vi "Sine Wave Test UI.vi"() -> ()   [LabVIEW 2015]
uses:
  Sub VIs/Actions.ctl
  Sub VIs/UI Refs.ctl
panel:
  in  "Help":bool
  in  "Settings":bool
  in  "Acquire":bool
  in  "Save":bool
  in  "Print":bool
  in  "Collapse Left":bool
  out "System Waveform Graph":dynamicdata(graph)=[{"t0"=timestamp(0 s since 1904-01-01), "dt"=0.001, "Y"=[-0.05212445512283584, -0.13336150644145808, 0.09686939475676047, 0.04269824059040653, 0.408386715636668, 0.1440963615851781, 0.18338040046154938, 0.5892398993428211, 0.2874755098028772, 0.42360867723351825, 0.39872198705884654, 0.49492986038483694, 0.8476469048510542, 0.5502130098060466, 0.7615388502014413, 0.6858061725246473, 0.765626496308488, 0.759950609248319, 0.913326650050298, 0.9293117069210004, 0.800454971802382, 0.9582885119713533, 1.033746579420675, 1.1831812892834357, 1.131684751301113, 1.1552984321319346, 0.9307610879266989, 1.0357903353668672, 0.7799760446349399, 0.9991309011630207, 0.9067651709329292, 0.9151844666347541, 0.7255708379595651, 0.7577153828467509, 0.76888934319496, 0.8791263479599363, 0.573195316103824, 0.82990628981861, 0.7959395065048407, 0.5455011585933895, 0.4133382261196344, 0.6023069220593702, 0.5471975645283245, 0.5729824629790687, 0.32581411586728487, 0.4323793250489525, 0.13206589194170887, 0.1566622503107214, 0.1943338680098371, -0.04642694048796602, -0.2187165688160441, -0.20901733138094658, 0.007409387766718373, -0.0945831190430492, -0.43328760979874337, -0.25787051409192135, -0.35671739178910694, -0.547611159639428, -0.7119832109077749, -0.6863088159770322, -0.7090502155660231, -0.7901918000137165, -0.6345319422588895, -0.8506202480018857, -0.952891386251698, -0.8864875433466509, -0.8104299150902663, -0.9655915717801792, -0.8044911508280994, -1.0556240415291098, -1.0702070678506619, -1.0265709175924453, -0.9505910211913751, -0.8618792724066139, -0.8436551316564458, -1.1601036667952578, -0.8804024988738188, -0.9488727250175957, -1.0109560414740402, -0.8017015754829107, -0.7668685893134745, -0.893413883311738, -0.7879424291614304, -0.8969827648567197, -0.6349738094147083, -0.592324080467644, -0.5406421151081083, -0.5744385812404026, -0.5106203917953414, -0.5414315844140066, -0.6483405504809772, -0.4993822273028547, -0.6243011215873379, -0.2714483922916202, -0.12038060671565365, -0.19885740767232296, -0.3350758453632484, -0.055660662182264856, -0.1953685024576336, -0.06497850198814607], "attributes"=variant("NI_ChannelName"=variant(string "Sine with Uniform Noise"), "NI_ExpIsRelativeTime"=variant(bool TRUE), "NI_ExpStartTimeStamp"=variant(timestamp timestamp(3347556890.3866034 s since 1904-01-01)), "NI_ExpTimeStamp"=variant(timestamp timestamp(3347556890.3866034 s since 1904-01-01)), "NI_ExpXDimension"=variant(string "t"))}, {"t0"=timestamp(0 s since 1904-01-01), "dt"=0.001, "Y"=[nan, nan, nan, nan, nan, nan, nan, nan, nan, nan, nan, nan, nan, nan, nan, nan, nan, nan, nan, nan, nan, nan, 1.033746579420675, 1.1831812892834357, 1.131684751301113, 1.1552984321319346, nan, 1.0357903353668672, nan, nan, nan, nan, nan, nan, nan, nan, nan, nan, nan, nan, nan, nan, nan, nan, nan, nan, nan, nan, nan, nan, nan, nan, nan, nan, nan, nan, nan, nan, nan, nan, nan, nan, nan, nan, nan, nan, nan, nan, nan, -1.0556240415291098, -1.0702070678506619, -1.0265709175924453, nan, nan, nan, -1.1601036667952578, nan, nan, -1.0109560414740402, nan, nan, nan, nan, nan, nan, nan, nan, nan, nan, nan, nan, nan, nan, nan, nan, nan, nan, nan, nan, nan], "attributes"=variant("NI_ChannelName"=variant(string "Failures"))}, {"t0"=timestamp(0 s since 1904-01-01), "dt"=0.001, "Y"=[1.0, 1.0, 1.0, 1.0, 1.0, 1.0, 1.0, 1.0, 1.0, 1.0, 1.0, 1.0, 1.0, 1.0, 1.0, 1.0, 1.0, 1.0, 1.0, 1.0, 1.0, 1.0, 1.0, 1.0, 1.0, 1.0, 1.0, 1.0, 1.0, 1.0, 1.0, 1.0, 1.0, 1.0, 1.0, 1.0, 1.0, 1.0, 1.0, 1.0, 1.0, 1.0, 1.0, 1.0, 1.0, 1.0, 1.0, 1.0, 1.0, 1.0, 1.0, 1.0, 1.0, 1.0, 1.0, 1.0, 1.0, 1.0, 1.0, 1.0, 1.0, 1.0, 1.0, 1.0, 1.0, 1.0, 1.0, 1.0, 1.0, 1.0, 1.0, 1.0, 1.0, 1.0, 1.0, 1.0, 1.0, 1.0, 1.0, 1.0, 1.0, 1.0, 1.0, 1.0, 1.0, 1.0, 1.0, 1.0, 1.0, 1.0, 1.0, 1.0, 1.0, 1.0, 1.0, 1.0, 1.0, 1.0, 1.0, 1.0], "attributes"=variant("NI_ChannelName"=variant(string "Upper Limit"))}, {"t0"=timestamp(0 s since 1904-01-01), "dt"=0.001, "Y"=[-1.0, -1.0, -1.0, -1.0, -1.0, -1.0, -1.0, -1.0, -1.0, -1.0, -1.0, -1.0, -1.0, -1.0, -1.0, -1.0, -1.0, -1.0, -1.0, -1.0, -1.0, -1.0, -1.0, -1.0, -1.0, -1.0, -1.0, -1.0, -1.0, -1.0, -1.0, -1.0, -1.0, -1.0, -1.0, -1.0, -1.0, -1.0, -1.0, -1.0, -1.0, -1.0, -1.0, -1.0, -1.0, -1.0, -1.0, -1.0, -1.0, -1.0, -1.0, -1.0, -1.0, -1.0, -1.0, -1.0, -1.0, -1.0, -1.0, -1.0, -1.0, -1.0, -1.0, -1.0, -1.0, -1.0, -1.0, -1.0, -1.0, -1.0, -1.0, -1.0, -1.0, -1.0, -1.0, -1.0, -1.0, -1.0, -1.0, -1.0, -1.0, -1.0, -1.0, -1.0, -1.0, -1.0, -1.0, -1.0, -1.0, -1.0, -1.0, -1.0, -1.0, -1.0, -1.0, -1.0, -1.0, -1.0, -1.0, -1.0], "attributes"=variant("NI_ChannelName"=variant(string "Lower Limit"))}]
  in  "Collapse Right":bool
  out "Table Control":string[][](table)=[["12/31/1903 6:00:00 PM", "-0.052"], ["12/31/1903 6:00:00 PM", "-0.133"], ["12/31/1903 6:00:00 PM", "0.097"], ["12/31/1903 6:00:00 PM", "0.043"], ["12/31/1903 6:00:00 PM", "0.408"], ["12/31/1903 6:00:00 PM", "0.144"], ["12/31/1903 6:00:00 PM", "0.183"], ["12/31/1903 6:00:00 PM", "0.589"], ["12/31/1903 6:00:00 PM", "0.287"], ["12/31/1903 6:00:00 PM", "0.424"], ["12/31/1903 6:00:00 PM", "0.399"], ["12/31/1903 6:00:00 PM", "0.495"], ["12/31/1903 6:00:00 PM", "0.848"], ["12/31/1903 6:00:00 PM", "0.550"], ["12/31/1903 6:00:00 PM", "0.762"], ["12/31/1903 6:00:00 PM", "0.686"], ["12/31/1903 6:00:00 PM", "0.766"], ["12/31/1903 6:00:00 PM", "0.760"], ["12/31/1903 6:00:00 PM", "0.913"], ["12/31/1903 6:00:00 PM", "0.929"], ["12/31/1903 6:00:00 PM", "0.800"], ["12/31/1903 6:00:00 PM", "0.958"], ["12/31/1903 6:00:00 PM", "1.034"], ["12/31/1903 6:00:00 PM", "1.183"], ["12/31/1903 6:00:00 PM", "1.132"], ["12/31/1903 6:00:00 PM", "1.155"], ["12/31/1903 6:00:00 PM", "0.931"], ["12/31/1903 6:00:00 PM", "1.036"], ["12/31/1903 6:00:00 PM", "0.780"], ["12/31/1903 6:00:00 PM", "0.999"], ["12/31/1903 6:00:00 PM", "0.907"], ["12/31/1903 6:00:00 PM", "0.915"], ["12/31/1903 6:00:00 PM", "0.726"], ["12/31/1903 6:00:00 PM", "0.758"], ["12/31/1903 6:00:00 PM", "0.769"], ["12/31/1903 6:00:00 PM", "0.879"], ["12/31/1903 6:00:00 PM", "0.573"], ["12/31/1903 6:00:00 PM", "0.830"], ["12/31/1903 6:00:00 PM", "0.796"], ["12/31/1903 6:00:00 PM", "0.546"], ["12/31/1903 6:00:00 PM", "0.413"], ["12/31/1903 6:00:00 PM", "0.602"], ["12/31/1903 6:00:00 PM", "0.547"], ["12/31/1903 6:00:00 PM", "0.573"], ["12/31/1903 6:00:00 PM", "0.326"], ["12/31/1903 6:00:00 PM", "0.432"], ["12/31/1903 6:00:00 PM", "0.132"], ["12/31/1903 6:00:00 PM", "0.157"], ["12/31/1903 6:00:00 PM", "0.194"], ["12/31/1903 6:00:00 PM", "-0.046"], ["12/31/1903 6:00:00 PM", "-0.219"], ["12/31/1903 6:00:00 PM", "-0.209"], ["12/31/1903 6:00:00 PM", "0.007"], ["12/31/1903 6:00:00 PM", "-0.095"], ["12/31/1903 6:00:00 PM", "-0.433"], ["12/31/1903 6:00:00 PM", "-0.258"], ["12/31/1903 6:00:00 PM", "-0.357"], ["12/31/1903 6:00:00 PM", "-0.548"], ["12/31/1903 6:00:00 PM", "-0.712"], ["12/31/1903 6:00:00 PM", "-0.686"], ["12/31/1903 6:00:00 PM", "-0.709"], ["12/31/1903 6:00:00 PM", "-0.790"], ["12/31/1903 6:00:00 PM", "-0.635"], ["12/31/1903 6:00:00 PM", "-0.851"], ["12/31/1903 6:00:00 PM", "-0.953"], ["12/31/1903 6:00:00 PM", "-0.886"], ["12/31/1903 6:00:00 PM", "-0.810"], ["12/31/1903 6:00:00 PM", "-0.966"], ["12/31/1903 6:00:00 PM", "-0.804"], ["12/31/1903 6:00:00 PM", "-1.056"], ["12/31/1903 6:00:00 PM", "-1.070"], ["12/31/1903 6:00:00 PM", "-1.027"], ["12/31/1903 6:00:00 PM", "-0.951"], ["12/31/1903 6:00:00 PM", "-0.862"], ["12/31/1903 6:00:00 PM", "-0.844"], ["12/31/1903 6:00:00 PM", "-1.160"], ["12/31/1903 6:00:00 PM", "-0.880"], ["12/31/1903 6:00:00 PM", "-0.949"], ["12/31/1903 6:00:00 PM", "-1.011"], ["12/31/1903 6:00:00 PM", "-0.802"], ["12/31/1903 6:00:00 PM", "-0.767"], ["12/31/1903 6:00:00 PM", "-0.893"], ["12/31/1903 6:00:00 PM", "-0.788"], ["12/31/1903 6:00:00 PM", "-0.897"], ["12/31/1903 6:00:00 PM", "-0.635"], ["12/31/1903 6:00:00 PM", "-0.592"], ["12/31/1903 6:00:00 PM", "-0.541"], ["12/31/1903 6:00:00 PM", "-0.574"], ["12/31/1903 6:00:00 PM", "-0.511"], ["12/31/1903 6:00:00 PM", "-0.541"], ["12/31/1903 6:00:00 PM", "-0.648"], ["12/31/1903 6:00:00 PM", "-0.499"], ["12/31/1903 6:00:00 PM", "-0.624"], ["12/31/1903 6:00:00 PM", "-0.271"], ["12/31/1903 6:00:00 PM", "-0.120"], ["12/31/1903 6:00:00 PM", "-0.199"], ["12/31/1903 6:00:00 PM", "-0.335"], ["12/31/1903 6:00:00 PM", "-0.056"], ["12/31/1903 6:00:00 PM", "-0.195"], ["12/31/1903 6:00:00 PM", "-0.065"]]
  in  "Cancel":bool
  out "Progress Bar":u8(slide) scale=0.0..100.0
  out "Status Bar Text":string="This is the status bar!"
  # "Sine Wave Tester"
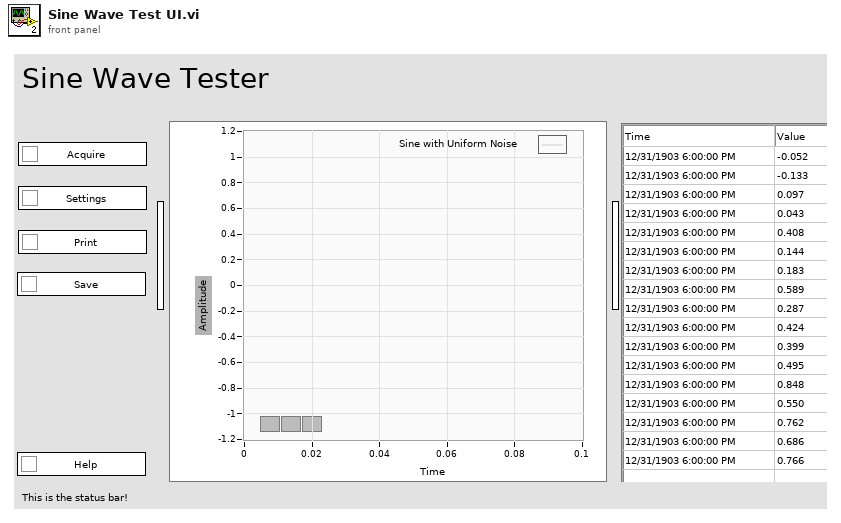
[diagram p1: front panel]
types:
  T1 = typedef "Actions.ctl" = enum16{"Help", "Panel Resize", "Print", "Settings", "Acquire", "Save"}
  T2 = cluster{"Select Printer":string, "Limit number of pages":dbl, "Filename":path, "Prompt for file path":bool, "When saving multiple files":enum32{"Radio Selection 1", "Radio Selection 2"}}
  T3 = typedef "UI Refs.ctl" = cluster{"Cancel Button Ref":refnum<vi>, "Status Bar Text Ref":refnum<vi>, "Progress Bar Ref":refnum<vi>, "This VI":refnum<vi>}
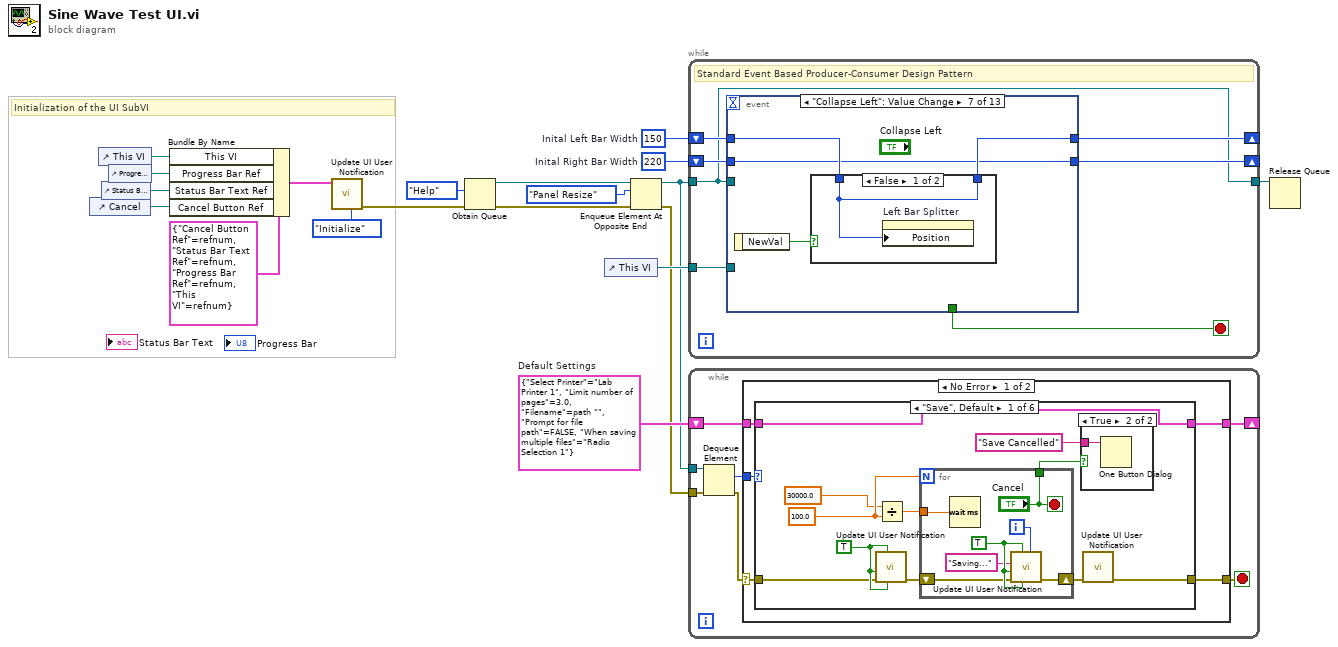
[diagram p0: block diagram]
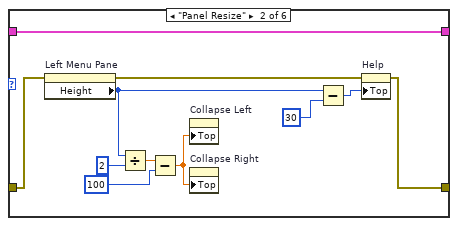
[diagram p3: hidden frame]
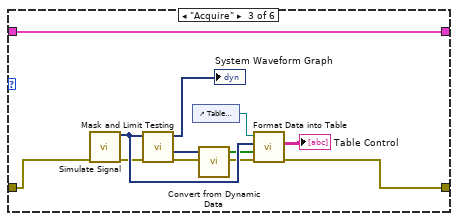
[diagram p4: hidden frame]
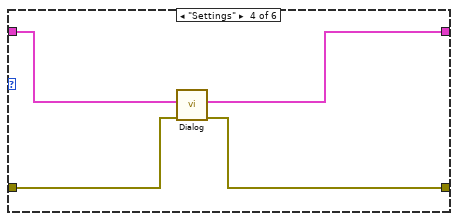
[diagram p5: hidden frame]
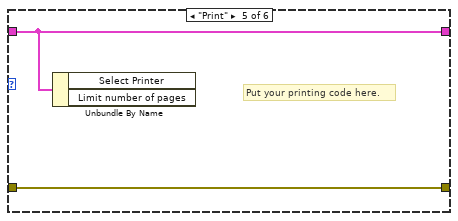
[diagram p6: hidden frame]
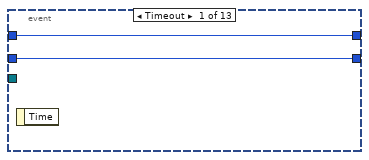
[diagram p9: hidden frame]
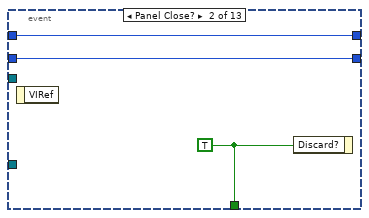
[diagram p10: hidden frame]
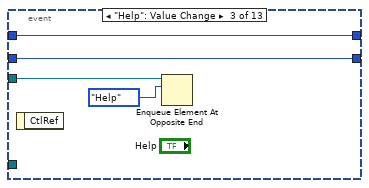
[diagram p11: hidden frame]
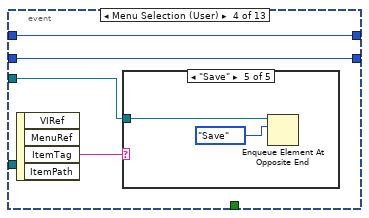
[diagram p12: hidden frame]
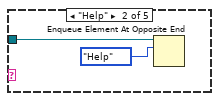
[diagram p14: hidden frame]
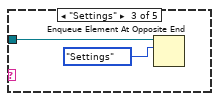
[diagram p15: hidden frame]
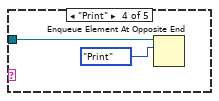
[diagram p16: hidden frame]
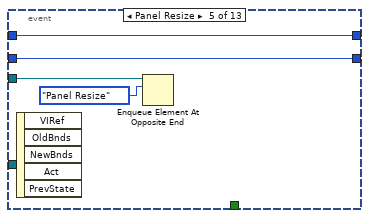
[diagram p17: hidden frame]
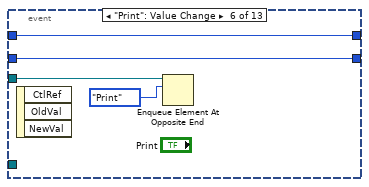
[diagram p18: hidden frame]
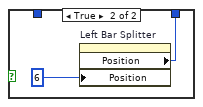
[diagram p19: hidden frame]
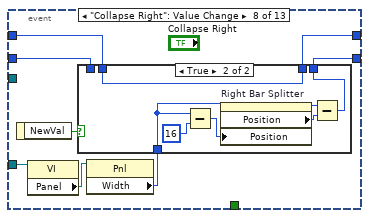
[diagram p20: hidden frame]
diagram:
  w7 = T2 {"Select Printer"="Lab Printer 1", "Limit number of pages"=3.0, "Filename"=path "", "Prompt for file path"=FALSE, "When saving multiple files"=enum."Radio Selection 1"}  # Default Settings
  w18 = 220  # Inital Right Bar Width
  w19 = 150  # Inital Left Bar Width
  # "Initialization of the UI SubVI"
  n1 = control-ref of="Cancel"() -> (w9:refnum<vi>)
  n2 = control-ref of="This VI"() -> (w12:refnum<vi>)
  n3 = control-ref of="Status Bar Text"() -> (w10:refnum<vi>)
  n4 = control-ref of="Progress Bar"() -> (w11:refnum<vi>)
  n5 = Bundle By Name(cluster=T3 {"Cancel Button Ref"=refnum, "Status Bar Text Ref"=refnum, "Progress Bar Ref"=refnum, "This VI"=refnum} ("UI Refs In"), "This VI"=w12, "Progress Bar Ref"=w11, "Status Bar Text Ref"=w10, "Cancel Button Ref"=w9) -> (w8:T3)
  n6 = call "Update UI User Notification.vi"("Action"=enum16{"Reset", "Set", "Initialize"}."Initialize", "UI Refs In"=w8) -> ("Error Out"=w6:errorcluster)  [unwired: 8 in, 1 out]
  n7 = Obtain Queue(element data type=Actions."Help" ("Enum"), error in (no error)=w6) -> (queue out=w5:refnum<queue>, error out=w2:errorcluster)  [unwired: 3 in, 1 out]
  n8 = control-ref of="This VI"() -> (w17:refnum<vi>)
  n9 = Enqueue Element At Opposite End(queue=w5, element=Actions."Panel Resize" ("Enum"), error in (no error)=w2) -> (queue out=w4:refnum<queue>, error out=w3:errorcluster)  [unwired: 1 in, 1 out]
  n10 = while {
    shift-right: [w23] -> _
    shift-left: w19 -> [w26]
    shift-right: [w22] -> _
    shift-left: w18 -> [w21]
    tunnel: w17 -> [w24]
    tunnel: w4 -> [w20]
    tunnel: [w20] -> w16
    stop <- w25 stop-if-true
    # "Standard Event Based Producer-Consumer Design Pattern"
    n11 = event shown="[6] \"Collapse Left\": Value Change" {
      selector: _ -> [_ _ _ _ _ _ _ _ _ _ _ _ _]
      dyn-events: _ -> [_ _ _ _ _ _ _ _ _ _ _ _ _]
      timeout: _ -> [_ _ _ _ _ _ _ _ _ _ _ _ _]
      tunnel: w26 -> [w28 w30 w35 w39 w51 w55 w57 w68 w83 w86 w89 w93 w97]
      tunnel: [w28 w30 w35 w39 w51 w55 w58 w69 w83 w86 w89 w93 w97] -> w23
      tunnel: [_ w31 _ _ _ _ _ _ _ _ _ _ _] -> w25
      tunnel: w24 -> [_ _ _ _ _ _ _ w67 _ _ _ _ _]
      tunnel: [w27 w29 w34 w38 w50 w54 w56 w64 w82 w85 w88 w92 w96] -> w22
      tunnel: w21 -> [w27 w29 w34 w38 w50 w54 w56 w63 w82 w85 w88 w92 w96]
      tunnel: w20 -> [_ _ w32 w36 w49 w52 _ _ _ _ w87 w94 w98]
      event Timeout {
        n12 = event-data() -> ()  [unwired: 1 in, 1 out]
      }
      event Panel Close? {
        w31 = TRUE ("Discard?")
        n13 = event-data() -> ()  [unwired: 1 in, 1 out]
        n14 = event-data("Discard?"=w31) -> ()  [unwired: 1 in, 1 out]
      }
      event "Help": Value Change {
        n15 = event-data() -> ()  [unwired: 1 in, 1 out]
        n16 = Enqueue Element At Opposite End(queue=w32, element=Actions."Help" ("Enum")) -> ()  [unwired: 2 in, 3 out]
      }
      event Menu Selection (User) {
        n17 = event-data() -> ("ItemTag"=w37:string)  [unwired: 1 in, 3 out]
        n18 = case shown="\"Save\"" w37 {
          tunnel: w36 -> [_ w41 w43 w45 w47]
          frame "False", Default {
          }
          frame "Help" {
            n19 = Enqueue Element At Opposite End(queue=w41, element=Actions."Help" ("Enum")) -> ()  [unwired: 2 in, 3 out]
          }
          frame "Settings" {
            n20 = Enqueue Element At Opposite End(queue=w43, element=Actions."Settings" ("Enum")) -> ()  [unwired: 2 in, 3 out]
          }
          frame "Print" {
            n21 = Enqueue Element At Opposite End(queue=w45, element=Actions."Print" ("Enum")) -> ()  [unwired: 2 in, 3 out]
          }
          frame "Save" {
            n22 = Enqueue Element At Opposite End(queue=w47, element=Actions."Save" ("Enum")) -> ()  [unwired: 2 in, 3 out]
          }
        }
      }
      event Panel Resize {
        n23 = event-data() -> ()  [unwired: 1 in, 5 out]
        n24 = Enqueue Element At Opposite End(queue=w49, element=Actions."Panel Resize" ("Enum")) -> ()  [unwired: 2 in, 3 out]
      }
      event "Print": Value Change {
        n25 = event-data() -> ()  [unwired: 1 in, 3 out]
        n26 = Enqueue Element At Opposite End(queue=w52, element=Actions."Print" ("Enum")) -> ()  [unwired: 2 in, 3 out]
      }
      event "Collapse Left": Value Change {
        n27 = event-data() -> ("NewVal"=w59:bool)  [unwired: 1 in]
        n28 = case shown="False" w59 {
          tunnel: [w60 w61] -> w58
          tunnel: w57 -> [w60 _]
          frame False {
            n29 = property on="Left Bar Splitter" class="Splitter"("Position"=w60) -> ()  [unwired: 2 in, 2 out]
          }
          frame True {
            n30 = property on="Left Bar Splitter" class="Splitter"("Position"=6 ("Splitter Position")) -> ("Position"=w61:i32)  [unwired: 2 in, 2 out]
          }
        }
      }
      event "Collapse Right": Value Change {
        n31 = event-data() -> ("NewVal"=w70:bool)  [unwired: 1 in]
        n32 = property class="VI"(reference=w67) -> ("Panel"=w66:refnum<vi>)  [unwired: 1 in, 2 out]
        n33 = property class="Pnl"(reference=w66) -> ("Width"=w65:u32)  [unwired: 1 in, 2 out]
        n34 = case shown="True" w70 {
          tunnel: [w74 w78] -> w69
          tunnel: w68 -> [w74 w78]
          tunnel: w65 -> [w72 w76]
          tunnel: [w71 w75] -> w64
          tunnel: w63 -> [w71 _]
          frame False {
            n35 = Subtract(x=w72, y=w71) -> (x-y=w73:u32)
            n36 = property on="Right Bar Splitter" class="Splitter"("Position"=w73) -> ()  [unwired: 2 in, 2 out]
          }
          frame True {
            n37 = Subtract(x=w76, y=16 ("Splitter Position")) -> (x-y=w79:u32)
            n38 = property on="Right Bar Splitter" class="Splitter"("Position"=w79) -> ("Position"=w77:i32)  [unwired: 2 in, 2 out]
            n39 = Subtract(x=w76, y=w77) -> (x-y=w75:u32)
          }
        }
      }
      event "Help", "Settings", "Acquire", "Save", "Print": Mouse Enter {
        n40 = event-data() -> ("CtlRef"=w84:refnum<vi>)  [unwired: 1 in]
        n41 = property class="Bool"(reference=w84) -> ("TipStrip"=w81:string)  [unwired: 1 in, 2 out]
        n42 = call "Update UI User Notification.vi"("Status Bar (\"\")"=w81) -> ()  [unwired: 9 in, 2 out]
      }
      event "Help", "Settings", "Acquire", "Save", "Print": Mouse Leave {
        # "The mouse left a mouseover item, reset the status bar"
        n43 = event-data() -> ()  [unwired: 1 in, 1 out]
        n44 = call "Update UI User Notification.vi"() -> ()  [unwired: 10 in, 2 out]
      }
      event "Settings": Value Change {
        n45 = event-data() -> ()  [unwired: 1 in, 1 out]
        n46 = Enqueue Element At Opposite End(queue=w87, element=Actions."Settings" ("Enum")) -> ()  [unwired: 2 in, 3 out]
      }
      event "Save": Value Change {
        n47 = event-data() -> ()  [unwired: 1 in, 1 out]
        n48 = Enqueue Element At Opposite End(queue=w94, element=Actions."Save" ("Enum")) -> ()  [unwired: 2 in, 3 out]
      }
      event "Acquire": Value Change {
        n49 = event-data() -> ()  [unwired: 1 in, 1 out]
        n50 = Enqueue Element At Opposite End(queue=w98, element=Actions."Acquire" ("Enum")) -> ()  [unwired: 2 in, 3 out]
      }
    }
  }
  n51 = while {
    tunnel: w4 -> [w105]
    tunnel: w3 -> [w101]
    shift-right: [w100] -> _
    shift-left: w7 -> [w99]
    stop <- w102 stop-if-true
    n52 = Dequeue Element(queue=w105, error in (no error)=w101) -> (element=w103:T1, error out=w104:errorcluster)  [unwired: 1 in, 2 out]
    n53 = case shown="No Error" w104 {
      selector: w104 -> [w109 w161]
      tunnel: w103 -> [w110 _]
      tunnel: [w108 w161] -> w102
      tunnel: [w107 w160] -> w100
      tunnel: w99 -> [w106 w160]
      frame No Error {
        n54 = case shown="\"Save\", Default" w110 {
          tunnel: w109 -> [w114 w136 w144 w155 w157 w159]
          tunnel: [w112 w135 w142 w154 w157 w159] -> w108
          tunnel: [w111 w140 w141 w153 w156 w158] -> w107
          tunnel: w106 -> [w111 w140 w141 w152 w156 w158]
          frame "Save", Default {
            w117 = TRUE ("Go")
            w121 = 100.0 ("y")
            n55 = call "Update UI User Notification.vi"("Cancel Visibile? (F)"=w117, "Progress Bar Visibile? (F)"=w117, "Error In"=w114, "Busy Cursor? (F)"=w117) -> ("Error Out"=w116:errorcluster)  [unwired: 6 in, 1 out]
            n56 = Divide(x=30000.0 ("y"), y=w121) -> (x/y=w120:dbl)
            n57 = for {
              N: w121 -> [_]
              tunnel: w120 -> [w129]
              tunnel: ["Cancel"] -> w119
              shift-right: [w123] -> w115
              shift-left: w116 -> [w124]
              i -> [w127]
              stop <- "Cancel" stop-if-true
              w126 = TRUE ("Go")
              n58 = Wait (ms)(milliseconds to wait=w129) -> ()  [unwired: 1 out]
              n59 = call "Update UI User Notification.vi"("Progress Bar Value (0)"=w127, "Cancel Visibile? (F)"=w126, "Progress Bar Visibile? (F)"=w126, "Error In"=w124, "Busy Cursor? (F)"=w126, "Status Bar (\"\")"="Saving..." ("Status Bar Text 2")) -> ("Error Out"=w123:errorcluster)  [unwired: 4 in, 1 out]
            }
            n60 = case shown="True" w119 {
              tunnel: "Save Cancelled" ("Status Bar Text 2") -> [_ w122]
              frame False {
              }
              frame True {
                n61 = One Button Dialog(message=w122) -> ()  [unwired: 1 in, 1 out]
              }
            }
            n62 = call "Update UI User Notification.vi"("Error In"=w115) -> ("Error Out"=w112:errorcluster)  [unwired: 9 in, 1 out]
          }
          frame "Panel Resize" {
            n63 = property on="Left Menu Pane" class="Pane"(error in=w136) -> (error out=w137:errorcluster, "Height"=w134:u32)  [unwired: 1 in, 1 out]
            n64 = Divide(x=w134, y=u32 2) -> (x/y=w132:dbl)
            n65 = Subtract(x=w132, y=u32 100) -> (x-y=w130:dbl)
            n66 = property on="Collapse Left" class="Bool (strict)"("Top"=w130) -> ()  [unwired: 2 in, 2 out]
            n67 = property on="Collapse Right" class="Bool (strict)"("Top"=w130) -> ()  [unwired: 2 in, 2 out]
            n68 = Subtract(x=w134, y=u32 30) -> (x-y=w138:u32)
            n69 = property on="Help" class="Bool"(error in=w137, "Top"=w138) -> (error out=w135:errorcluster)  [unwired: 1 in, 1 out]
          }
          frame "Acquire" {
            n70 = call "Simulate Signal"("error in (no error)"=w144) -> ("Sine with Uniform Noise"=w151:dynamicdata, "error out"=w145:errorcluster)  [unwired: 13 in]
            n71 = call "Mask and Limit Testing"("error in"=w145, "Signals"=w151) -> ("error out"=w143:errorcluster, "Point Evaluation"=w146:dynamicdata, "Tested Signals"=→"System Waveform Graph":dynamicdata)  [unwired: 6 in, 1 out]
            n72 = control-ref of="Table Control"() -> (w149:refnum<vi>)
            n73 = call "Convert from Dynamic Data"("Dynamic Data Type"=w146) -> ("Array"=w147:bool[])  [unwired: 3 in]
            n74 = call "Format Data into Table.vi"("error in (no error)"=w143, "Passed?"=w147, "Signals"=w151, "Tbl Refnum"=w149) -> ("error out"=w142:errorcluster, "Table"=→"Table Control":string[][])  [unwired: 5 in, 1 out]
          }
          frame "Settings" {
            n75 = call "Dialog.vi"("error in (no error)"=w155, "Settings In"=w152) -> ("error out"=w154:errorcluster, "Settings Out"=w153:T2)  [unwired: 8 in]
          }
          frame "Print" {
            # "Put your printing code here."
            n76 = Unbundle By Name(w156) -> ()  [unwired: 2 out]
          }
          frame "Help" {
          }
        }
      }
      frame Error {
      }
    }
  }
  n77 = Release Queue(queue=w16) -> ()  [unwired: 2 in, 3 out]
